vi "writeAttributesToFile.vi"(0 "HGF_IMAQDevice":refnum<class "HGF_IMAQDevice.lvclass">, 2 "Filename":path, 5 "error in (no error)":errorcluster) -> (14 "dup HGF_IMAQDevice":refnum<class "HGF_IMAQDevice.lvclass">, 19 "error out":errorcluster)   [LabVIEW 2014, in "HGF_IMAQ.lvlib" / "HGF_IMAQDevice.lvclass"]
doc: "Saves a configuration file for a camera."
uses:
  HGF_IMAQDevice.lvclass
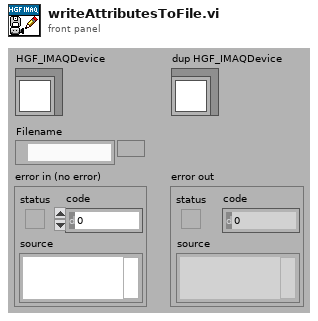
[diagram p1: front panel]
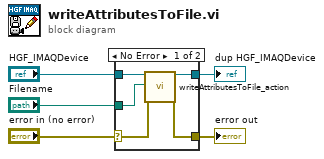
[diagram p0: block diagram]
diagram:
  n1 = case shown="No Error" "error in (no error)" {
    selector: "error in (no error)" -> [w8 w12]
    tunnel: [w7 w12] -> w4
    tunnel: [w9 w11] -> w2
    tunnel: "HGF_IMAQDevice" -> [w10 w11]
    tunnel: "Filename" -> [w6 _]
    frame No Error {
      n2 = call-dynamic "writeAttributesToFile_action.vi"("HGF_IMAQDevice"=w10, "Filename"=w6, "error in (no error)"=w8) -> ("dup HGF_IMAQDevice"=w9:refnum<class "HGF_IMAQDevice.lvclass">, "error out"=w7:errorcluster)  [unwired: 15 in]
    }
    frame Error {
    }
  }
  "error out" <- w4
  "dup HGF_IMAQDevice" <- w2
